vi "MainTagBrowser.vi"() -> ()   [LabVIEW 2013]
doc: "Read Binary File opens and reads an existing file stored as a double precision array in binary form. This VI shows the simplest way to read this entire file, with the simplest error checking."
panel:
  out "TagValue":string
  out "TagName":string
  out "TagType":string
  in  "Tag_num":i32 min=0 max=0
  out "n_hdr_items":i32=80
  out "file error status":errorcluster
  out "Version":string
  out "Magic":string
  # "Select the tag number here and see the content below"
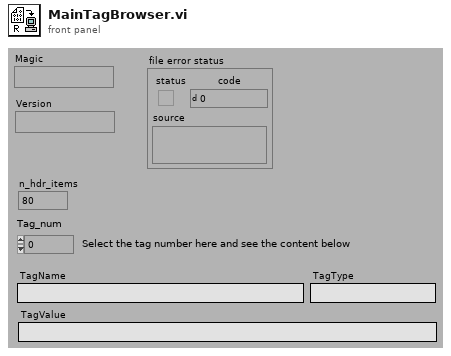
[diagram p1: front panel]
types:
  T1 = cluster{"TagIdent":string, "TagIndex":i32, "TagType":i32, "TagValue":i64, "TagAuxData":string}
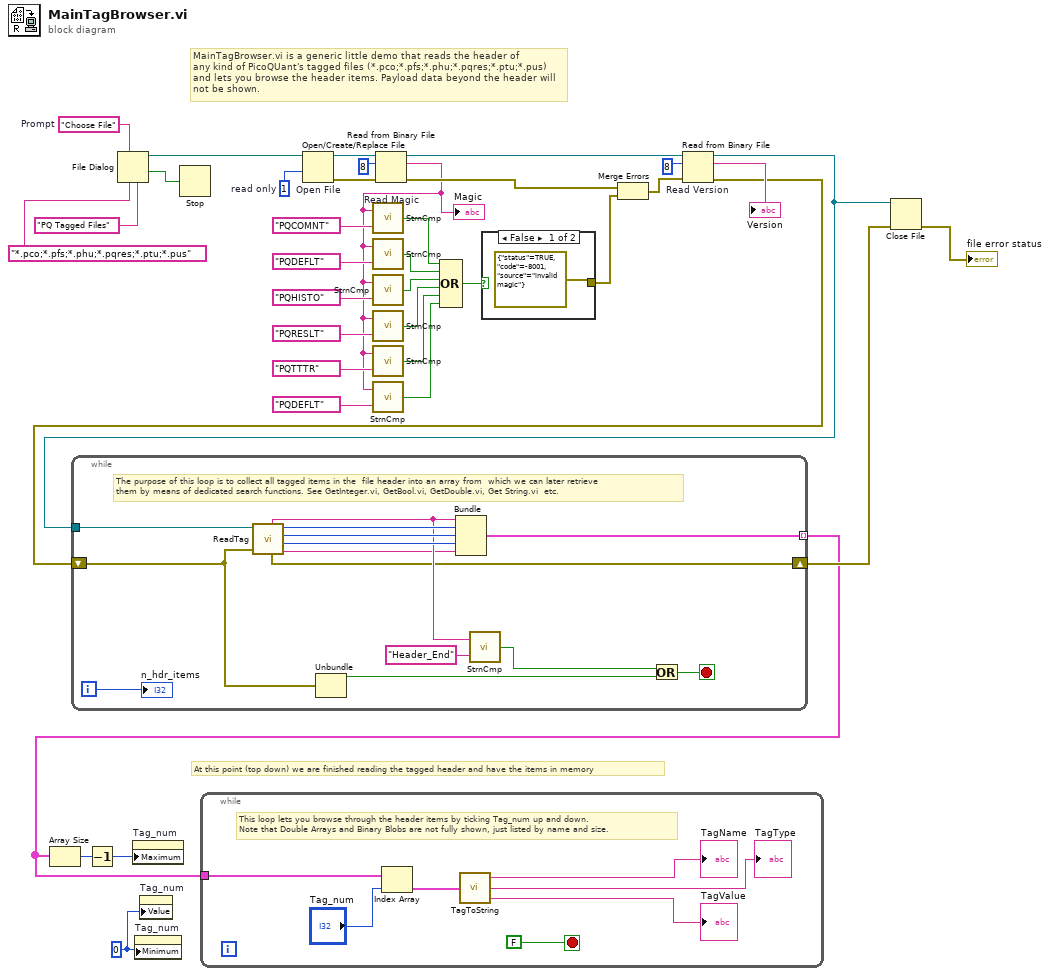
[diagram p0: block diagram]
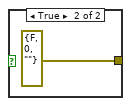
[diagram p2: hidden frame]
diagram:
  w2 = 0
  w1 = 1  # read only
  w36 = "Choose File"  # Prompt
  # "MainTagBrowser.vi is a generic little demo that reads the header of\nany kind of PicoQUant's tagged files (*.pco;*.pfs;*.phu;*.pqres;*.ptu;*.pus)\nand lets you browse the header items. Payload data beyond the header will \nnot be shown."
  # "At this point (top down) we are finished reading the tagged header and have the items in memory"
  n1 = File Dialog(4:"PQ Tagged Files", 6:"*.pco;*.pfs;*.phu;*.pqres;*.ptu;*.pus", 7:w36) -> (1:w24:bool, 3:w37:path)  [unwired: 4 in, 2 out]
  n2 = property on="Tag_num" class="DigNum (strict)"("Minimum"=w2) -> ()  [unwired: 2 in, 2 out]
  n3 = property on="Tag_num" class="DigNum (strict)"("Value"=w2) -> ()  [unwired: 2 in, 2 out]
  n4 = Stop(stop? (T)=w24) -> ()
  n5 = Open/Create/Replace File "Open File"(file path (use dialog)=w37, access (0:read/write)=w1) -> (refnum out=w26:refnum<file>, error out=w25:errorcluster)  [unwired: 4 in, 1 out]
  n6 = Read from Binary File "Read Magic"(8:w25, 10:8, 11:w26) -> (0:w30:errorcluster, 2:w6:string, 3:w35:refnum<file>)  [unwired: 3 in, 1 out]
  "Magic" <- w6
  n7 = call "StrnCmp.vi"("String 2"="PQCOMNT", "String 1"=w6) -> ("equal"=w13:bool)
  n8 = call "StrnCmp.vi"("String 2"="PQDEFLT", "String 1"=w6) -> ("equal"=w12:bool)
  n9 = call "StrnCmp.vi"("String 2"="PQHISTO", "String 1"=w6) -> ("equal"=w11:bool)
  n10 = call "StrnCmp.vi"("String 2"="PQRESLT", "String 1"=w6) -> ("equal"=w10:bool)
  n11 = call "StrnCmp.vi"("String 2"="PQTTTR", "String 1"=w6) -> ("equal"=w9:bool)
  n12 = call "StrnCmp.vi"("String 2"="PQDEFLT", "String 1"=w6) -> ("equal"=w8:bool)
  n13 = Compound Arithmetic op=OR(w13, w12, w11, w10, w9, w8) -> (w7:bool)
  n14 = case shown="False" w7 {
    tunnel: [errorcluster {"status"=TRUE, "code"=-8001, "source"="invalid magic"} ("file error status 2") errorcluster {"status"=FALSE, "code"=0, "source"=""} ("file error status 2")] -> w28
    frame False {
    }
    frame True {
    }
  }
  n15 = Merge Errors(w30, w28) -> (w29:errorcluster)
  n16 = Read from Binary File "Read Version"(8:w29, 10:8, 11:w35) -> (0:w23:errorcluster, 2:→"Version":string, 3:w21:refnum<file>)  [unwired: 3 in, 1 out]
  n17 = while {
    shift-left: w23 -> [w51]
    shift-right: [w40] -> w22
    tunnel: w21 -> [w53]
    tunnel: [w47] -> w5 mode=indexing
    i -> [w46]
    stop <- w52 stop-if-true
    # "The purpose of this loop is to collect all tagged items in the  file header into an array from  which we can later retrieve \nthem by means of dedicated search functions. See GetInteger.vi, GetBool.vi, GetDouble.vi, Get String.vi  etc."
    n18 = call "ReadTag.vi"("refnum"=w53, "error in"=w51) -> ("TagIdent"=w42:string, "TagIndex"=w50:i32, "TagType"=w49:i32, "error out"=w40:errorcluster, "TagValue"=w48:i64, "TagAuxData"=w41:string)  [unwired: 3 in]
    n19 = Unbundle(w51) -> ("status"=w43:bool)  [unwired: 2 out]
    n20 = Bundle("TagIdent"=w42, "TagIndex"=w50, "TagType"=w49, "TagValue"=w48, "TagAuxData"=w41) -> (w47:T1)  [unwired: 1 in]
    n21 = call "StrnCmp.vi"("String 2"="Header_End", "String 1"=w42) -> ("equal"=w44:bool)
    n22 = Or(x=w44, y=w43) -> (x .or. y?=w52:bool)
    "n_hdr_items" <- w46
  }
  n23 = Array Size(array=w5) -> (size(s)=w4:i32)
  n24 = Decrement(x=w4) -> (x-1=w3:i32)
  n25 = property on="Tag_num" class="DigNum (strict)"("Maximum"=w3) -> ()  [unwired: 2 in, 2 out]
  n26 = while {
    tunnel: w5 -> [w59]
    stop <- FALSE stop-if-true
    # "This loop lets you browse through the header items by ticking Tag_num up and down.\nNote that Double Arrays and Binary Blobs are not fully shown, just listed by name and size."
    n27 = Index Array(array=w59, index="Tag_num") -> (element=w57:T1)
    n28 = call "TagToString.vi"("TagData"=w57) -> ("StrTagValue"=→"TagValue":string, "StrTagType"=→"TagType":string, "StrTagName"=→"TagName":string)  [unwired: 2 in]
  }
  n29 = Close File(refnum=w21, error in=w22) -> (error out=→"file error status":errorcluster)  [unwired: 1 out]
